vi "Find Particle.vi"(7 "File Path":path, 8 "error in":errorcluster, 9 "Camera Image":T2, 10 "From File":bool, 11 "R/G/B":cluster{"Lower value":i32, "Upper value":i32}[](array[cluster])) -> (0 "error out":errorcluster, 1 "Circles":T1(array[cluster]) {"Position"."Y" format="%.2f"; "Position"."X" format="%.2f"}, 2 "Thresholded Image":T2(plugin-control), 3 "Base Image":T2(plugin-control), 5 "Number of Particles":i32)   [LabVIEW 2016]
uses:
  <vilib>/vision/Image Controls.llb/IMAQ Image.ctl
  <vilib>/vision/NI_Vision_Development_Module.lvlib
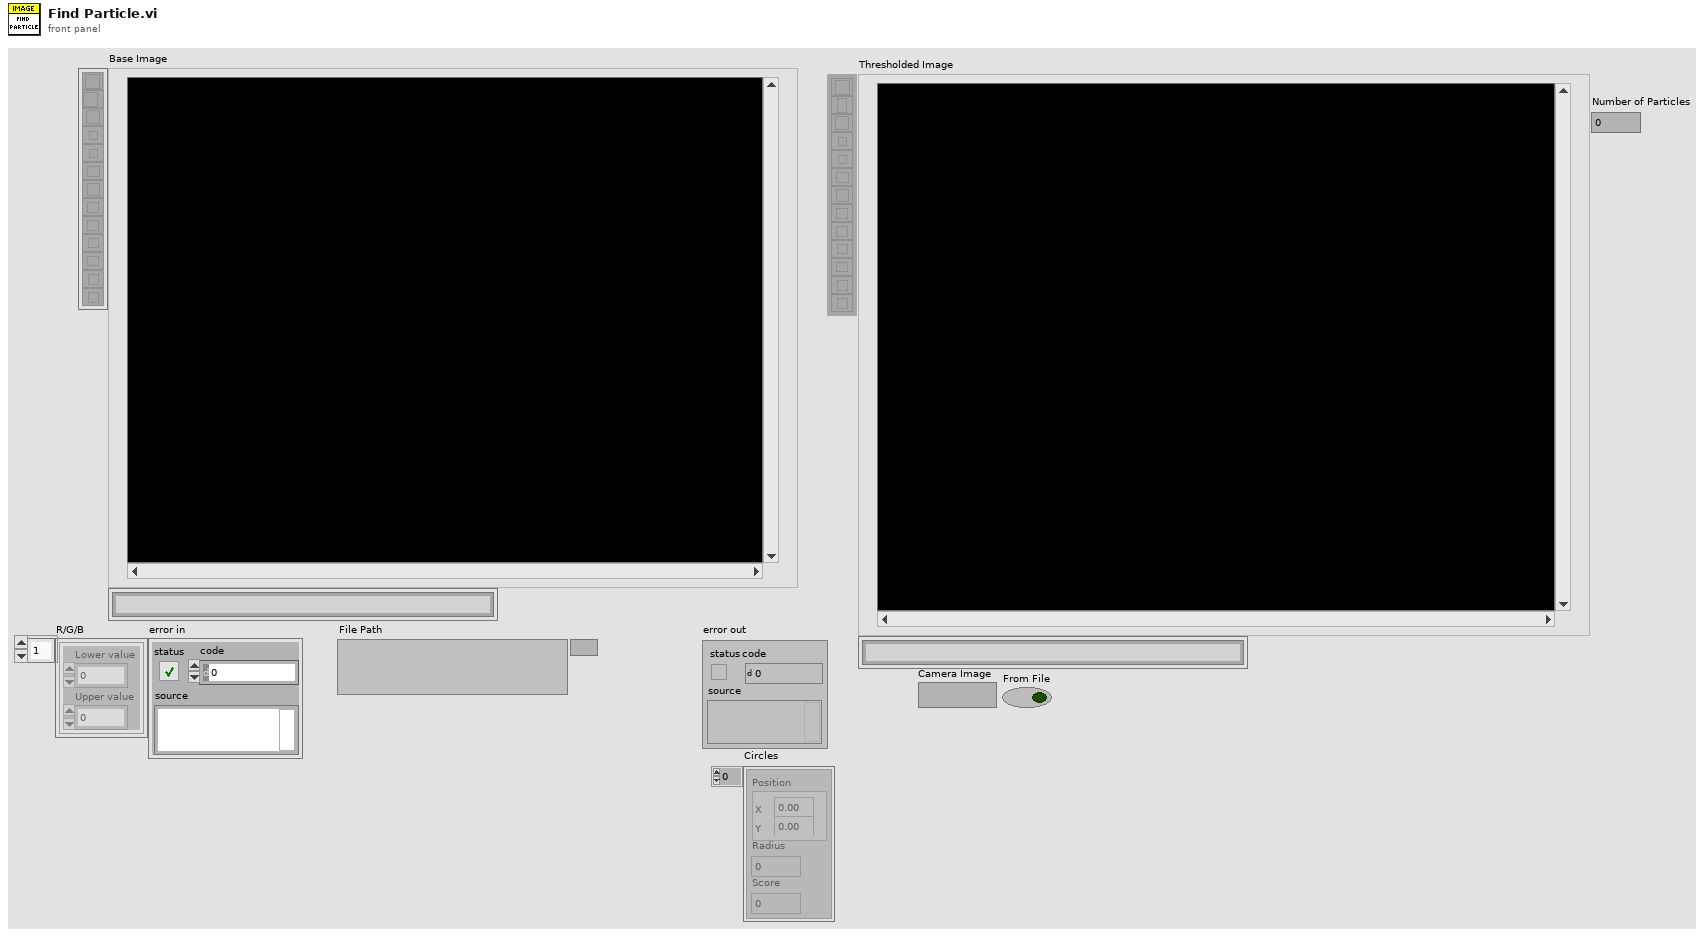
[diagram p1: front panel]
types:
  T1 = cluster{"Position":cluster{"X":sgl, "Y":sgl}, "Radius":dbl, "Score":dbl}[]
  T2 = typedef "IMAQ Image.ctl" = refnum<image>
  T3 = typedef "Image Type" = u32
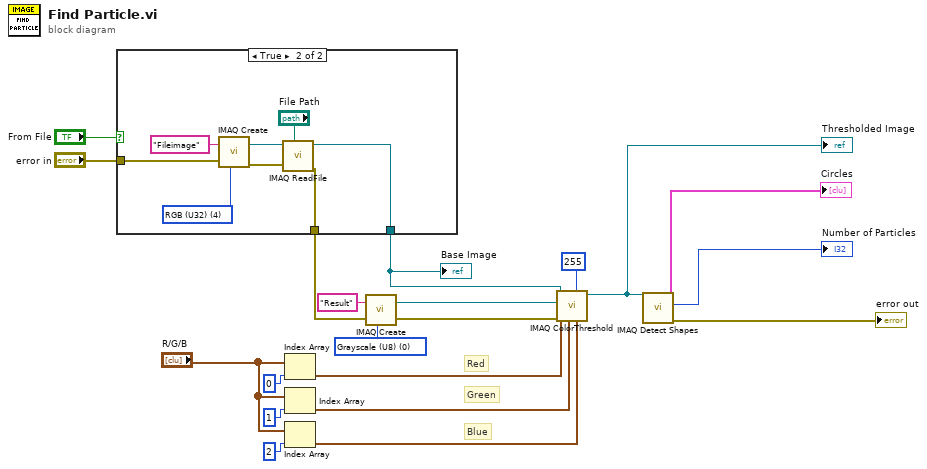
[diagram p0: block diagram]
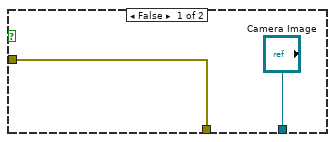
[diagram p2: hidden frame]
diagram:
  w19 = T3 0 items=["Grayscale (U8)", "Grayscale (I16)", "Grayscale (SGL)", "Complex (CSG)", "RGB (U32)", "HSL (U32)", "RGB (U64)", "Grayscale (U16)"] ("Image Type")
  # "Blue"
  # "Green"
  # "Red"
  n1 = case shown="True" "From File" {
    tunnel: ["Camera Image" w26] -> w9
    tunnel: [w21 w25] -> w6
    tunnel: "error in" -> [w21 w24]
    frame False {
    }
    frame True {
      w28 = T3 4 items=["Grayscale (U8)", "Grayscale (I16)", "Grayscale (SGL)", "Complex (CSG)", "RGB (U32)", "HSL (U32)", "RGB (U64)", "Grayscale (U16)"] ("Image Type")
      n2 = call "IMAQ Create"("Image Name"="Fileimage", "Image Type"=w28, "error in (no error)"=w24) -> ("New Image"=w30:T2, "error out"=w29:errorcluster)  [unwired: 2 in]
      n3 = call "IMAQ ReadFile"("File Path"="File Path", "error in (no error)"=w29, "Image"=w30) -> ("error out"=w25:errorcluster, "Image Out"=w26:T2)  [unwired: 4 in, 3 out]
    }
  }
  "Base Image" <- w9
  n4 = Index Array(array="R/G/B", index=0) -> (element=w12:cluster{"Lower value":i32, "Upper value":i32})
  n5 = Index Array(array="R/G/B", index=1) -> (element=w11:cluster{"Lower value":i32, "Upper value":i32})
  n6 = Index Array(array="R/G/B", index=2) -> (element=w10:cluster{"Lower value":i32, "Upper value":i32})
  n7 = call "IMAQ Create"("Image Name"="Result", "Image Type"=w19, "error in (no error)"=w6) -> ("New Image"=w18:T2, "error out"=w7:errorcluster)  [unwired: 2 in]
  n8 = call "IMAQ ColorThreshold"("Blue or Luma or Val or Inten Range"=w10, "Replace Value"=255, "Green or Sat Range"=w11, "error in (no error)"=w7, "Red or Hue Range"=w12, "Image Dst"=w18, "Image Src"=w9) -> ("Image Dst Out"=w3:T2)  [unwired: 3 in, 1 out]
  "Thresholded Image" <- w3
  n9 = call-poly "IMAQ Detect Shapes"("Image"=w3) -> ("error out"=→"error out":errorcluster, "Number of Matches Returned"=→"Number of Particles":i32, "Circles"=→"Circles":T1)  [unwired: 8 in]
